vi "Proportional Stabilization.vi"() -> ()   [LabVIEW 2013]
uses:
  Global Variables/Global Stop.vi
panel:
  out "Thin Etalon Pos Setp on Activation":i32
  in  "Thin Etalon Position Setpoint":i32
  in  "Etalon Selection":enum16{"Thick Etalon", "Thin Etalon"}(ring)
  in  "Activate Output":bool
  out "Thick Etalon Pos Setp on Activation":i32
  out "Wavenumber on Activation":dbl format="%.4f"
  in  "Correction Output":bool
  out "correction steps":dbl
  in  "Difference Threshold":dbl=0.019999999999999997
  in  "Proportional Correction Factor":dbl=300.0
  out "New Wavemeter Value":bool
  out "Out of Range":bool
  in  "Stop":bool
  out "Loop Counter":i32
  in  "Thick Etalon Position Setpoint":i32
  in  "Invert Output":bool
  in  "Wavenumber Setpoint":dbl format="%.4f"
  out "Wavenumber Acquisition":dbl format="%.4f"
  # "Invert Output\nif moving beyond\nFlash Position"
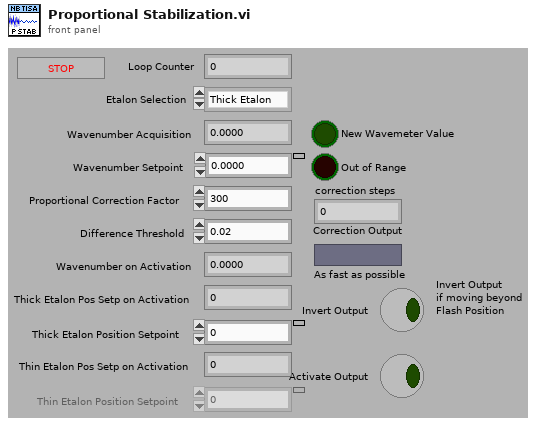
[diagram p1: front panel]
types:
  T1 = enum8{"Enabled", "Disabled", "Disabled and Grayed Out"}
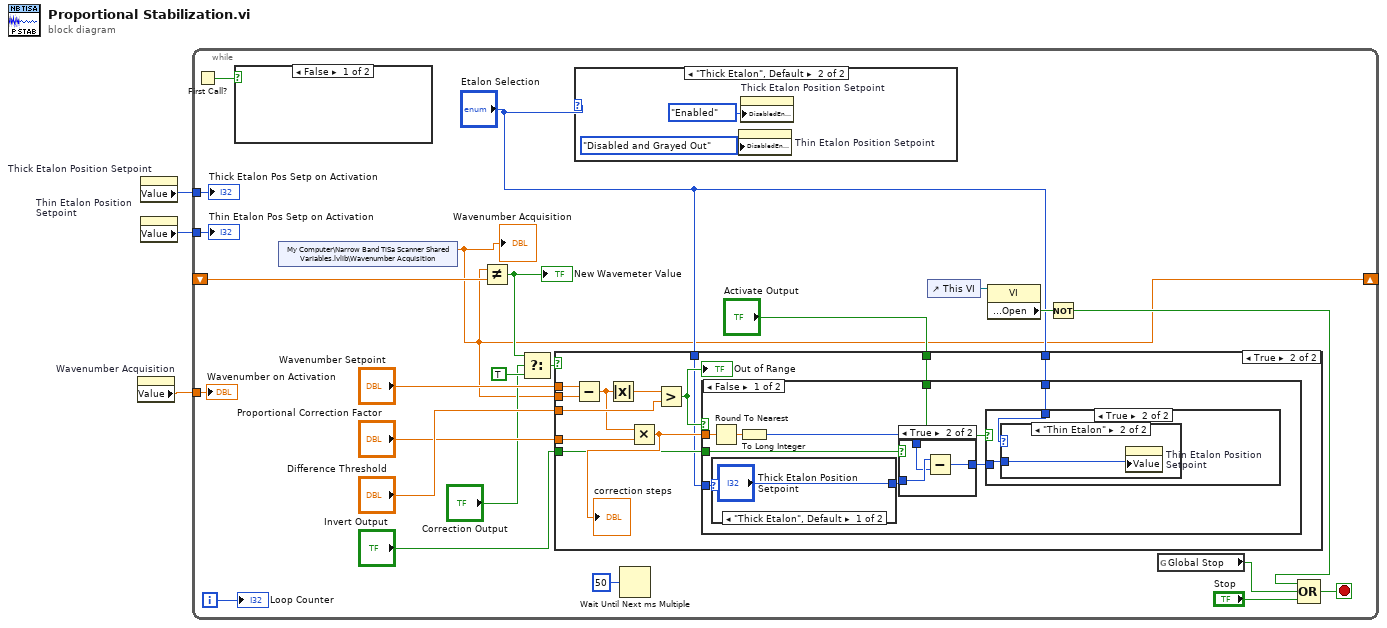
[diagram p0: block diagram]
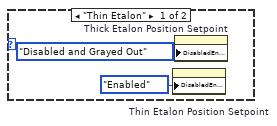
[diagram p2: hidden frame]
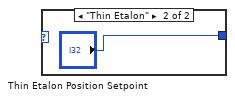
[diagram p4: hidden frame]
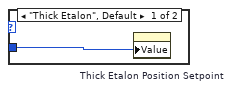
[diagram p6: hidden frame]
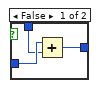
[diagram p7: hidden frame]
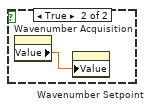
[diagram p9: hidden frame]
diagram:
  n1 = property on="Wavenumber Acquisition" class="DigNum (strict)"() -> ("Value"=w3:dbl)  [unwired: 2 in, 2 out]
  n2 = property on="Thick Etalon Position Setpoint" class="DigNum (strict)"() -> ("Value"=w2:i32)  [unwired: 2 in, 2 out]
  n3 = property on="Thin Etalon Position Setpoint" class="DigNum (strict)"() -> ("Value"=w1:i32)  [unwired: 2 in, 2 out]
  n4 = while {
    shift-right: [w4] -> _
    shift-left: _ -> [w26]
    tunnel: w3 -> [w9]
    tunnel: w2 -> [w8]
    tunnel: w1 -> [w6]
    i -> [w23]
    stop <- w13 stop-if-true
    n5 = First Call?() -> (First Call?: T/F=w27:bool)
    n6 = case shown="False" w27 {
      frame False {
      }
      frame True {
        n7 = property on="Wavenumber Acquisition" class="DigNum (strict)"() -> ("Value"=w65:dbl)  [unwired: 2 in, 2 out]
        n8 = property on="Wavenumber Setpoint" class="DigNum (strict)"("Value"=w65) -> ()  [unwired: 2 in, 2 out]
      }
    }
    n9 = shared-variable "My Computer\\Narrow Band TiSa Scanner Shared Variables.lvlib\\Wavenumber Acquisition"() -> (w4:dbl)  [unwired: 1 in, 1 out]
    "Wavenumber Acquisition" <- w4
    n10 = Not Equal?(x=w4, y=w26) -> (x != y?=w18:bool)
    "New Wavemeter Value" <- w18
    n11 = Select(t=w18, s="Correction Output", f=TRUE) -> (s? t:f=w19:bool)
    n12 = case shown="True" w19 {
      tunnel: "Wavenumber Setpoint" -> [_ w43]
      tunnel: w4 -> [_ w42]
      tunnel: "Difference Threshold" -> [_ w39]
      tunnel: "Proportional Correction Factor" -> [_ w37]
      tunnel: "Invert Output" -> [_ w35]
      tunnel: "Activate Output" -> [_ w34]
      tunnel: "Etalon Selection" -> [_ w33]
      tunnel: "Etalon Selection" -> [_ w32]
      frame False {
      }
      frame True {
        n13 = Subtract(x=w43, y=w42) -> (x-y=w38:dbl)
        n14 = Absolute Value(x=w38) -> (abs(x)=w41:dbl)
        n15 = Multiply(x=w38, y=w37) -> (x*y=w36:dbl)
        "correction steps" <- w36
        n16 = Greater?(x=w41, y=w39) -> (0:w40:bool)
        "Out of Range" <- w40
        n17 = case shown="False" w40 {
          tunnel: w36 -> [w51 _]
          tunnel: w35 -> [w49 _]
          tunnel: w34 -> [w46 _]
          tunnel: w33 -> [w45 _]
          tunnel: w32 -> [w44 _]
          frame False {
            n18 = Round To Nearest(number=w51) -> (nearest integer value=w48:dbl)
            n19 = case shown="\"Thick Etalon\", Default" w44 {
              tunnel: ["Thick Etalon Position Setpoint" "Thin Etalon Position Setpoint"] -> w52
              frame "Thick Etalon", Default {
              }
              frame "Thin Etalon" {
              }
            }
            n20 = To Long Integer(number=w48) -> (32bit integer=w47:i32)
            n21 = case shown="True" w49 {
              tunnel: w52 -> [w61 w64]
              tunnel: w47 -> [w60 w63]
              tunnel: [w59 w62] -> w50
              frame False {
                n22 = Add(x=w61, y=w60) -> (x+y=w59:i32)
              }
              frame True {
                n23 = Subtract(x=w64, y=w63) -> (x-y=w62:i32)
              }
            }
            n24 = case shown="True" w46 {
              tunnel: w50 -> [_ w56]
              tunnel: w45 -> [_ w55]
              frame False {
              }
              frame True {
                n25 = case shown="\"Thin Etalon\"" w55 {
                  tunnel: w56 -> [w57 w58]
                  frame "Thick Etalon", Default {
                    n26 = property on="Thick Etalon Position Setpoint" class="DigNum (strict)"("Value"=w57) -> ()  [unwired: 2 in, 2 out]
                  }
                  frame "Thin Etalon" {
                    n27 = property on="Thin Etalon Position Setpoint" class="DigNum (strict)"("Value"=w58) -> ()  [unwired: 2 in, 2 out]
                  }
                }
              }
            }
          }
          frame True {
          }
        }
      }
    }
    n28 = case shown="\"Thick Etalon\", Default" "Etalon Selection" {
      frame "Thin Etalon" {
        n29 = property on="Thin Etalon Position Setpoint" class="DigNum (strict)"("DisabledEnum"=T1."Enabled" ("Disabled")) -> ()  [unwired: 2 in, 2 out]
        n30 = property on="Thick Etalon Position Setpoint" class="DigNum (strict)"("DisabledEnum"=T1."Disabled and Grayed Out" ("Disabled")) -> ()  [unwired: 2 in, 2 out]
      }
      frame "Thick Etalon", Default {
        n31 = property on="Thin Etalon Position Setpoint" class="DigNum (strict)"("DisabledEnum"=T1."Disabled and Grayed Out" ("Disabled")) -> ()  [unwired: 2 in, 2 out]
        n32 = property on="Thick Etalon Position Setpoint" class="DigNum (strict)"("DisabledEnum"=T1."Enabled" ("Disabled")) -> ()  [unwired: 2 in, 2 out]
      }
    }
    n33 = Wait Until Next ms Multiple(millisecond multiple=u32 50) -> ()  [unwired: 1 out]
    n34 = control-ref of="This VI"() -> (w14:refnum<vi>)
    n35 = property class="VI"(reference=w14) -> ("Front Panel.Open"=w15:bool)  [unwired: 1 in, 2 out]
    n36 = Not(x=w15) -> (.not. x?=w12:bool)
    n37 = global read "Global Stop.vi" "Global Stop"() -> (w11:bool)
    n38 = Compound Arithmetic op=OR(w12, w11, "Stop") -> (w13:bool)
    "Loop Counter" <- w23
    "Wavenumber on Activation" <- w9
    "Thick Etalon Pos Setp on Activation" <- w8
    "Thin Etalon Pos Setp on Activation" <- w6
  }
